vi "类型3自动测试结果.vi"(8 "合格?":bool, 11 "第几组":i32) -> ()   [LabVIEW 2010]
uses:
  全局量/自动测试结果.vi
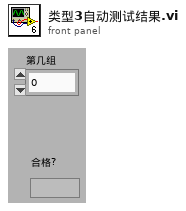
[diagram p1: front panel]
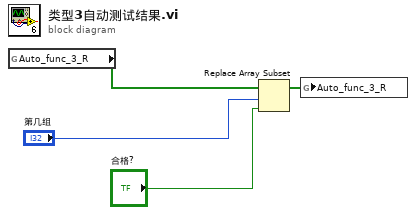
[diagram p0: block diagram]
diagram:
  n1 = global read "自动测试结果.vi" "Auto_func_3_R"() -> (w4:bool[])
  n2 = Replace Array Subset(array=w4, new element="合格?", index="第几组") -> (w3:bool[])
  n3 = global write "自动测试结果.vi" "Auto_func_3_R"(w3) -> ()
